vi "RunOperation.vi"(10 "Inputs":string[](array[string]), 11 "RunUnitTests in":refnum<class "RunUnitTests.lvclass">) -> (1 "Output/Failure":string, 2 "CLI Process Return Code":i32, 3 "RunUnitTests out":refnum<class "RunUnitTests.lvclass">)   [LabVIEW 2014, in "RunUnitTests.lvclass"]
uses:
  RunUnitTests.lvclass
panel:
  in  "Operation Output/Error Out":string="The RunUnitTests operation is not supported on Mac and Linux."
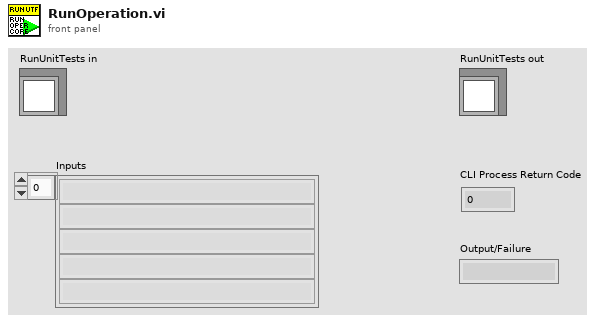
[diagram p1: front panel]
types:
  T1 = typedef "NI_UnitTestFramework.lvlib/utf_test_result_overall.ctl" = cluster{"utf results out":T2[], "untested VIs":cluster{"VI path":path, "code coverage":T11, "vi hierarchy":string[]}[], "project file path":path, "system information":string}
  T2 = typedef "NI_UnitTestFramework.lvlib/utf_test_result_testfile.ctl" = cluster{"test case":T3[], "test status":T4, "test path":path, "setup VI":path, "teardown VI":path, "code coverage":T11, "start time":timestamp, "end time":timestamp, "test hierarchy":string[], "VI path":path, "VI timestamp":timestamp, "VI rev hist":i32, "requirements ID":string, "array brackets":string, "name separator":string, "errors":T12[], "paragraph header":string, "result comment":string, "vi hierarchy":string[], "subVI coverage info":T11[], "subVI info":T14[], "big array threshold":u32, "VI Index":i32, "Comment":string, "Dynamic Dispatch":bool, "User-defined test VI":path, "user-defined VI code coverage":T11}
  T3 = typedef "NI_UnitTestFramework.lvlib/utf_test_result_testcase.ctl" = cluster{"test result":T4, "run Times":T5[], "test case name":string, "requirements":string, "code coverage":T11, "subVI coverage info":T11[]}
  T4 = typedef "NI_UnitTestFramework.lvlib/utf_test_result.ctl" = enum16{"Passed", "Failed", "Error", "Skipped", "Not Processed"}
  T5 = typedef "NI_UnitTestFramework.lvlib/utf_test_result_troll_new.ctl" = cluster{"result (test)":T4, "Vector Result":T6[]}
  T6 = typedef "NI_UnitTestFramework.lvlib/utf_vector_result.ctl" = cluster{"time elapsed [ms]":u32, "result (test)":T4, "result (parameters)":T7[], "Used Vector Values":cluster{"Vector Name":string, "element":i32}[], "Executed Class Path":path, "Input":T10[]}
  T7 = typedef "NI_UnitTestFramework.lvlib/utf_test_result_failure.ctl" = cluster{"result":T4, "error message":string, "parameter name":string, "parameter value":variant, "parameters":variant[], "comparison":T8, "requirement ID":string, "VI":T9, "Used Vector Name":string}
  T8 = typedef "NI_UnitTestFramework.lvlib/utf_test_comparison_operators.ctl" = enum16{"=", "!=", ">", ">=", "<", "<=", "range", "symmetric tolerance", "asymmetric tolerance", "string contains", "string not contain", "array size", "string length", "array range", "by element", "array range (limit array)", "user-defined", "array contains", "array not contain", "vector length", "= (elm)", "!= (elm)", "= (case insensitive)", "!= (case insensitive)"}
  T9 = typedef "NI_UnitTestFramework.lvlib/utf_vi_tag.ctl" = enum16{"Setup VI", "VI under Test", "Teardown VI"}
  T10 = typedef "NI_UnitTestFramework.lvlib/utf_test_result_input_data.ctl" = cluster{"Name":string, "Input Value":variant[], "VI":T9, "Used Vector Index":i32}
  T11 = typedef "NI_UnitTestFramework.lvlib/utf_code_coverage.ctl" = cluster{"coverage":dbl, "diagram run flag":bool[]}
  T12 = typedef "NI_UnitTestFramework.lvlib/utf_error_data.ctl" = cluster{"error type":T13, "description":string}
  T13 = typedef "NI_UnitTestFramework.lvlib/utf_error_type.ctl" = enum16{"TestFileError", "VIError", "SetupVIError", "TearDownVIError", "OtherError"}
  T14 = typedef "NI_UnitTestFramework.lvlib/utf_subvi_info.ctl" = cluster{"Path":path, "Dependence VI":bool}
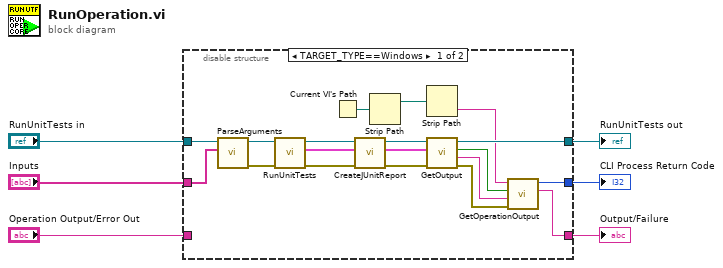
[diagram p0: block diagram]
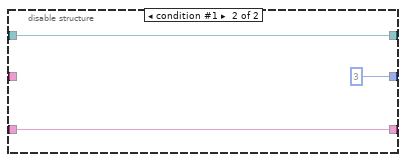
[diagram p2: hidden frame]
diagram:
  n1 = disable-structure shown="TARGET_TYPE==Windows" {
    disable-tunnel: "RunUnitTests in" -> [w25 w28]
    disable-tunnel: [w24 w28] -> w5
    disable-tunnel: "Inputs" -> [w23 _]
    disable-tunnel: [w11 3 ("CLI Process Return Code")] -> w3
    disable-tunnel: [w10 w26] -> w2
    disable-tunnel: "Operation Output/Error Out" -> [_ w26]
    frame condition #0 (active) {
      n2 = call-dynamic "ParseArguments.vi"("Inputs"=w23, "RunUnitTests in"=w25) -> ("error out"=w16:errorcluster, "RunUnitTests out"=w17:refnum<class "RunUnitTests.lvclass">)  [unwired: 8 in]
      n3 = call "RunUnitTests.vi"("error in (no error)"=w16, "RunUnitTests in"=w17) -> ("error out"=w21:errorcluster, "test results out"=w18:T1, "RunUnitTests out"=w22:refnum<class "RunUnitTests.lvclass">)  [unwired: 7 in]
      n4 = Current VI's Path() -> (path=w9:path)
      n5 = call "CreateJUnitReport.vi"("error in (no error)"=w21, "test results in"=w18, "RunUnitTests in"=w22) -> ("error out"=w20:errorcluster, "test results out"=w15:T1, "RunUnitTests out"=w19:refnum<class "RunUnitTests.lvclass">)  [unwired: 6 in]
      n6 = Strip Path(path=w9) -> (stripped path=w8:path)  [unwired: 1 out]
      n7 = Strip Path(path=w8) -> (name=w7:string)  [unwired: 1 out]
      n8 = call "GetOutput.vi"("error in (no error)"=w20, "test results in"=w15, "RunUnitTests in"=w19) -> ("error out"=w14:errorcluster, "Output"=w13:string, "Passed"=w12:bool, "RunUnitTests out"=w24:refnum<class "RunUnitTests.lvclass">)  [unwired: 5 in]
      n9 = call "GetOperationOutput.vi"("error in (no error)"=w14, "Operation Output/Error In"=w13, "Operation succeeded?"=w12, "Operation Name"=w7) -> ("Operation Output/Error Out"=w10:string, "CLI Process Return Code"=w11:i32)  [unwired: 6 in]
    }
    frame condition #1 {
    }
  }
  "RunUnitTests out" <- w5
  "CLI Process Return Code" <- w3
  "Output/Failure" <- w2
